vi "Init.vi"(8 "error in (no error)":errorcluster, 10 "Price":dbl, 11 "Couch in":refnum<class "Couch.lvclass">) -> (0 "error out":errorcluster, 3 "Couch out":refnum<class "Couch.lvclass">)   [LabVIEW 2019, in "Couch.lvclass"]
uses:
  Couch.lvclass
  Furniture.lvclass
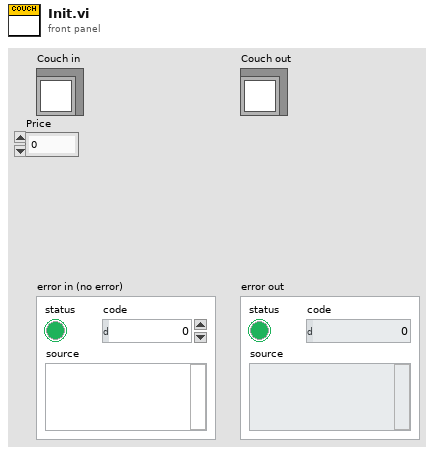
[diagram p1: front panel]
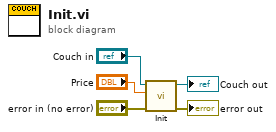
[diagram p0: block diagram]
diagram:
  n1 = call-parent "Init.vi"("error in (no error)"="error in (no error)", "Price"="Price", "Furniture in"="Couch in") -> ("error out"=→"error out":errorcluster, "Furniture out"=→"Couch out":refnum<class "Couch.lvclass">)  [unwired: 7 in]
